vi "ANC300_GetSerial.vi"(0 "ANC300 Communication Port In":refnum<visa-resource-name>, 1 "connection ID in":refnum<k5>, 3 "Axis":u16(ring) items=["Main", "Axis 1", "Axis 2", "Axis 3", "Axis 4", "Axis 5", "Axis 6", "Axis 7"], 5 "error in":T1, 7 "Time to wait [ms]":u32=200) -> (10 "command string":string, 13 "data out":string, 14 "ANC300 Communication Port Out":refnum<visa-resource-name>, 15 "connection ID out":refnum<k5>, 16 "transfer ok":bool, 17 "Serial":string, 18 "Serial OK":bool, 19 "error out":T1)   [LabVIEW 2023]
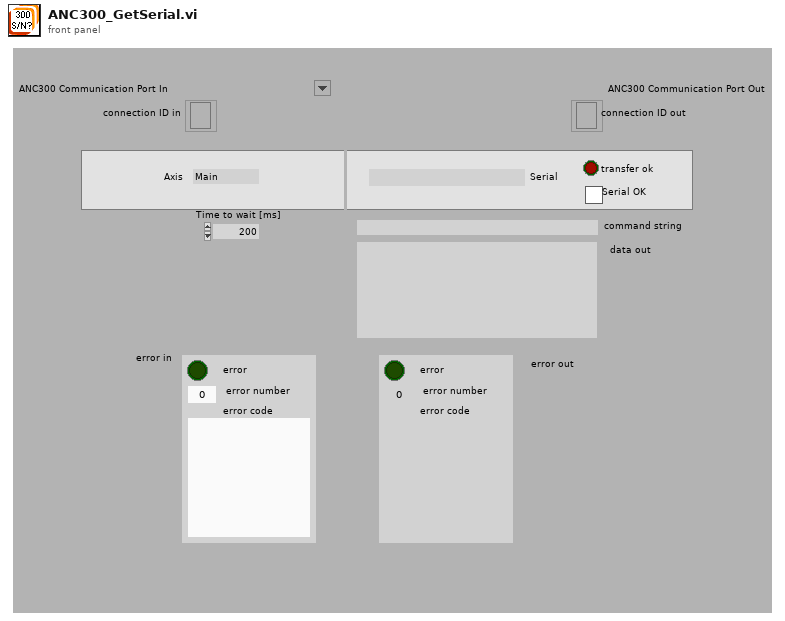
[diagram p1: front panel]
types:
  T1 = cluster{"error ":bool, "error number":i32, "error code":string}
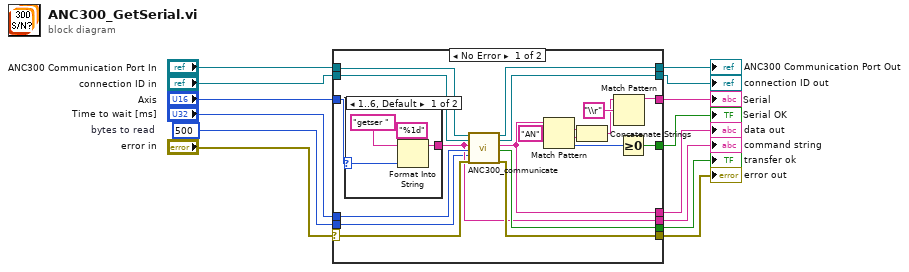
[diagram p0: block diagram]
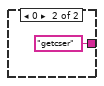
[diagram p2: hidden frame]
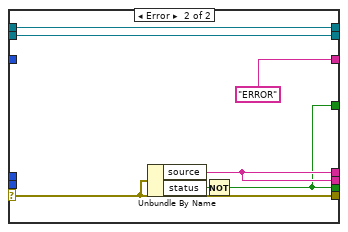
[diagram p3: hidden frame]
diagram:
  w11 = 500  # bytes to read
  n1 = case shown="No Error" "error in" {
    selector: "error in" -> [w29 w44]
    tunnel: "ANC300 Communication Port In" -> [w34 w46]
    tunnel: "connection ID in" -> [w33 w45]
    tunnel: "Time to wait [ms]" -> [w32 _]
    tunnel: w11 -> [w16 _]
    tunnel: [w31 w44] -> w5
    tunnel: [w15 w46] -> w9
    tunnel: [w30 w45] -> w8
    tunnel: [w28 w40] -> w4
    tunnel: [w27 w42] -> w7
    tunnel: [w17 w42] -> w6
    tunnel: "Axis" -> [w26 _]
    tunnel: [w18 "ERROR"] -> w2
    tunnel: [w21 w40] -> w1
    frame No Error {
      n2 = case shown="1..6, Default" w26 {
        selector: w26 -> [w35 _]
        tunnel: [w38 "getcser"] -> w27
        frame 1..6, Default {
          n3 = Format Into String(format string="%1d", initial string="getser ", w35) -> (resulting string=w38:string)  [unwired: 1 in, 1 out]
        }
        frame 0 {
        }
      }
      n4 = call "ANC300_communicate.vi"("ANC300 Communication Port In"=w34, "connection ID in"=w33, "commando string"=w27, "Time to wait [ms]"=w32, "bytes to read"=w16, "error in"=w29) -> ("ANC300 Communication Port Out"=w15:refnum<visa-resource-name>, "connection ID out"=w30:refnum<k5>, "read data"=w17:string, "transfer ok"=w28:bool, "error out"=w31:T1)  [unwired: 9 in]
      n5 = Match Pattern(string=w17, regular expression="AN") -> (match substring=w22:string, after substring=w23:string, offset past match=w24:i32)  [unwired: 1 in, 1 out]
      n6 = Concatenate Strings(w22, w23) -> (w19:string)
      n7 = Match Pattern(string=w19, regular expression="\\r") -> (before substring=w18:string)  [unwired: 1 in, 3 out]
      n8 = Greater Or Equal To 0?(x=w24) -> (x >= 0?=w21:bool)
    }
    frame Error {
      n9 = Unbundle By Name(w44) -> ("source"=w42:string, "status"=w43:bool)
      n10 = Not(x=w43) -> (.not. x?=w40:bool)
    }
  }
  "data out" <- w6
  "connection ID out" <- w8
  "error out" <- w5
  "command string" <- w7
  "transfer ok" <- w4
  "ANC300 Communication Port Out" <- w9
  "Serial" <- w2
  "Serial OK" <- w1
